vi "NanoValve VI.vi"(1 "Time to load sample":dbl, 2 "Time to hold in inject position (s)":dbl, 3 "Number of injections":dbl, 4 "VISA resource name":refnum<visa-resource-name>) -> (0 "Error Out":errorcluster)   [LabVIEW 2014]
uses:
  <vilib>/Instr/_visa.llb/VISA Configure Serial Port (Instr).vi
panel:
  in  "Stop/Start":bool
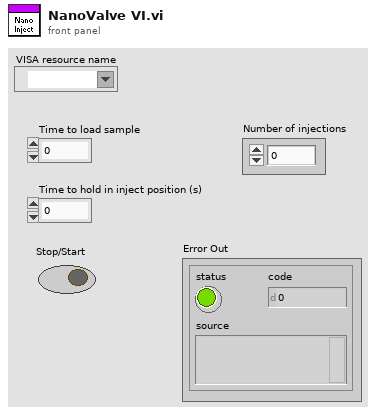
[diagram p1: front panel]
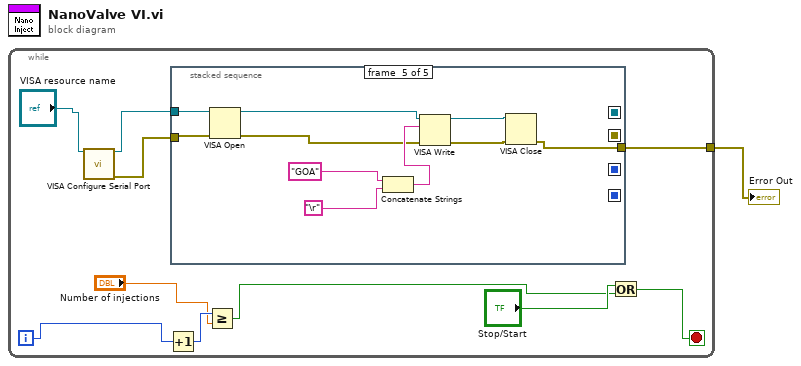
[diagram p0: block diagram]
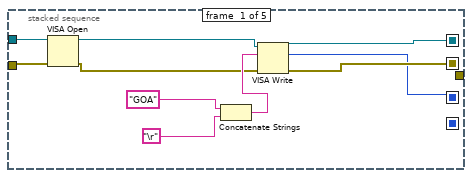
[diagram p2: hidden frame]
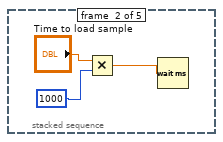
[diagram p3: hidden frame]
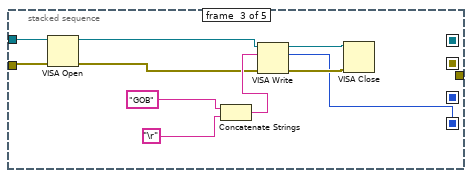
[diagram p4: hidden frame]
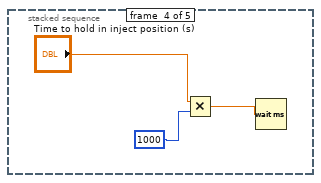
[diagram p5: hidden frame]
diagram:
  n1 = while {
    tunnel: [w2] -> w1
    i -> [w5]
    stop <- w6 stop-if-true
    n2 = call-poly "VISA Configure Serial Port"("VISA resource name"="VISA resource name") -> ("VISA resource name out"=w10:refnum<visa-resource-name>, "error out"=w9:errorcluster)  [unwired: 13 in]
    n3 = Increment(x=w5) -> (x+1=w4:i32)
    n4 = stacked-sequence {
      seq-local: [w15 _ _ _ _] -> [_ _ _ _ _]
      seq-local: [w14 _ _ _ _] -> [_ _ _ _ _]
      seq-local: [w13 _ _ _ _] -> [_ _ _ _ _]
      seq-local: [_ _ w27 _ _] -> [_ _ _ _ _]
      tunnel: w10 -> [w21 _ w34 _ w47]
      tunnel: w9 -> [w20 _ w33 _ w46]
      tunnel: [_ _ _ _ w38] -> w2
      frame #0 {
        n5 = VISA Open(error in (no error)=w20, VISA resource name=w21) -> (VISA resource name=w18:refnum<visa-resource-name>, error out=w16:errorcluster)  [unwired: 3 in]
        n6 = Concatenate Strings("GOA", "\r") -> (w17:string)
        n7 = VISA Write(VISA resource name=w18, write buffer=w17, error in (no error)=w16) -> (VISA resource name out=w15:refnum<visa-resource-name>, return count=w13:u32, error out=w14:errorcluster)
      }
      frame #1 {
        n8 = Multiply(x="Time to load sample", y=1000) -> (x*y=w23:dbl)
        n9 = Wait (ms)(milliseconds to wait=w23) -> ()  [unwired: 1 out]
      }
      frame #2 {
        n10 = VISA Open(error in (no error)=w33, VISA resource name=w34) -> (VISA resource name=w26:refnum<visa-resource-name>, error out=w25:errorcluster)  [unwired: 3 in]
        n11 = Concatenate Strings("GOB", "\r") -> (w30:string)
        n12 = VISA Write(VISA resource name=w26, write buffer=w30, error in (no error)=w25) -> (VISA resource name out=w29:refnum<visa-resource-name>, return count=w27:u32, error out=w28:errorcluster)
        n13 = VISA Close(VISA resource name=w29, error in (no error)=w28) -> ()  [unwired: 1 out]
      }
      frame #3 {
        n14 = Multiply(x="Time to hold in inject position (s)", y=1000) -> (x*y=w37:dbl)
        n15 = Wait (ms)(milliseconds to wait=w37) -> ()  [unwired: 1 out]
      }
      frame #4 {
        n16 = VISA Open(error in (no error)=w46, VISA resource name=w47) -> (VISA resource name=w40:refnum<visa-resource-name>, error out=w39:errorcluster)  [unwired: 3 in]
        n17 = Concatenate Strings("GOA", "\r") -> (w43:string)
        n18 = VISA Write(VISA resource name=w40, write buffer=w43, error in (no error)=w39) -> (VISA resource name out=w42:refnum<visa-resource-name>, error out=w41:errorcluster)  [unwired: 1 out]
        n19 = VISA Close(VISA resource name=w42, error in (no error)=w41) -> (error out=w38:errorcluster)
      }
    }
    n20 = Greater Or Equal?(x=w4, y="Number of injections") -> (x >= y?=w7:bool)
    n21 = Or(x="Stop/Start", y=w7) -> (x .or. y?=w6:bool)
  }
  "Error Out" <- w1
